vi "Configure Sampling Rate.vi"(8 "error in (no error)":errorcluster, 10 "Sample Rate (1000 Hz)":i32=1000, 11 "VISA resource name":refnum<visa-resource-name>) -> (0 "error out":errorcluster, 3 "VISA resource name out":refnum<visa-resource-name>)   [LabVIEW 2015, in "Micron Optics sm130.lvlib"]
doc: "Configures the sampling rate of the instrument in Hz. Be aware that the sampling rate is dependent on the wavelength range. The range cannot be configured by the user. Most instruments have an 80 nm wavelength range and so the max sampling rate is 1000 Hz. Instruments with a 40 nm wavelength range can have a sampling rate of upto 2 kHz."
uses:
  Micron Optics sm130.lvlib
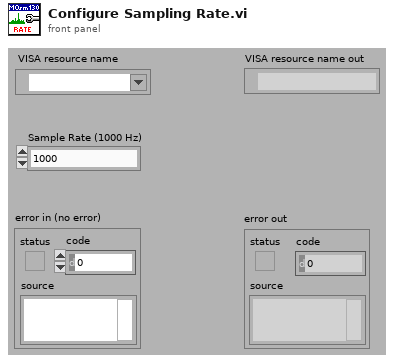
[diagram p1: front panel]
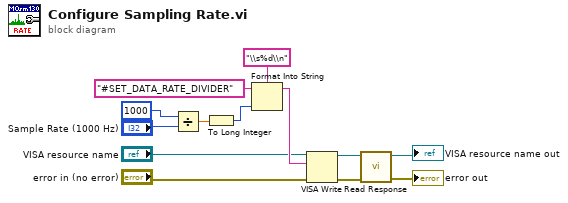
[diagram p0: block diagram]
diagram:
  n1 = Divide(x=1000, y="Sample Rate (1000 Hz)") -> (x/y=w4:dbl)
  n2 = To Long Integer(number=w4) -> (32bit integer=w3:i32)
  n3 = Format Into String(format string="\\s%d\\n", initial string="#SET_DATA_RATE_DIVIDER", w3) -> (resulting string=w11:string)  [unwired: 1 in, 1 out]
  n4 = VISA Write(VISA resource name="VISA resource name", write buffer=w11, error in (no error)="error in (no error)") -> (VISA resource name out=w10:refnum<visa-resource-name>, error out=w9:errorcluster)  [unwired: 1 out]
  n5 = call "Read Response.vi"("error in (no error)"=w9, "VISA resource name"=w10) -> ("error out"=→"error out":errorcluster, "VISA resource name out"=→"VISA resource name out":refnum<visa-resource-name>)  [unwired: 7 in, 1 out]
